vi "Blink.vi"(11 "Port":enum8{"ONE", "TWO"}(ring)) -> (3 "ByteArrayToSend":u8[](array[numeric]) format="%x")   [LabVIEW 2019]
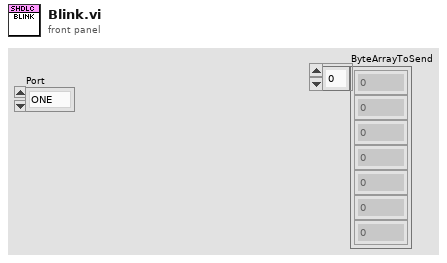
[diagram p1: front panel]
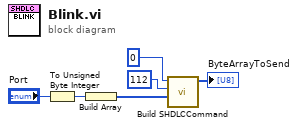
[diagram p0: block diagram]
diagram:
  n1 = To Unsigned Byte Integer(number="Port") -> (unsigned 8bit integer=w3:u8)
  n2 = Build Array(w3) -> (w2:u8[])
  n3 = call "Build SHDLCCommand.vi"("Data"=w2, "CommandID"=u8 112, "SlaveAdress"=u8 0) -> ("ByteArrayToSend"=→"ByteArrayToSend":u8[])  [unwired: 8 in]
